vi "InitializePicomotor8742Controller.vi"(8 "error in (no error)":errorcluster, 11 "Picomotor8742 in":refnum<class "Picomotor8742.lvclass">) -> (0 "error out":errorcluster, 3 "Picomotor8742 out":refnum<class "Picomotor8742.lvclass">)   [LabVIEW 2020, in "Picomotor8742.lvclass"]
doc: "Initialize the class \"Picomotor8742ControllerClass\" that handles the communication with the physical device , and open the communication with the device"
uses:
  Picomotor8742.lvclass
  SupportLibs/TCPCommClass/TCPCommClass.lvclass
  C:/GEECS/Developers Version/source/Device Drivers/Picomotor8742/SupportLibs/ASCIICommClass/ASCIICommClass.lvclass
  SupportLibs/PicoMotorController/Picomoto8742ControllerClass.lvclass
  SupportLibs/PicoMotor8472Comm/PicoMotor8742Comm.lvclass
  Picomotor8742.lvclass/Picomotor8742.ctl
  SupportLibs/PicoMotor8742Axis/Picomotor8742Axis.lvclass
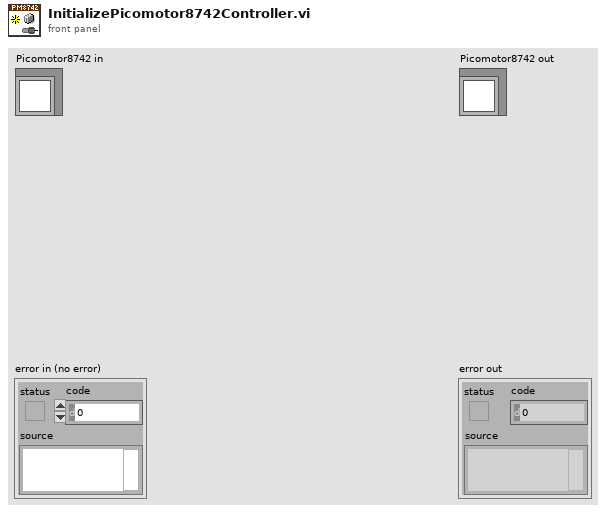
[diagram p1: front panel]
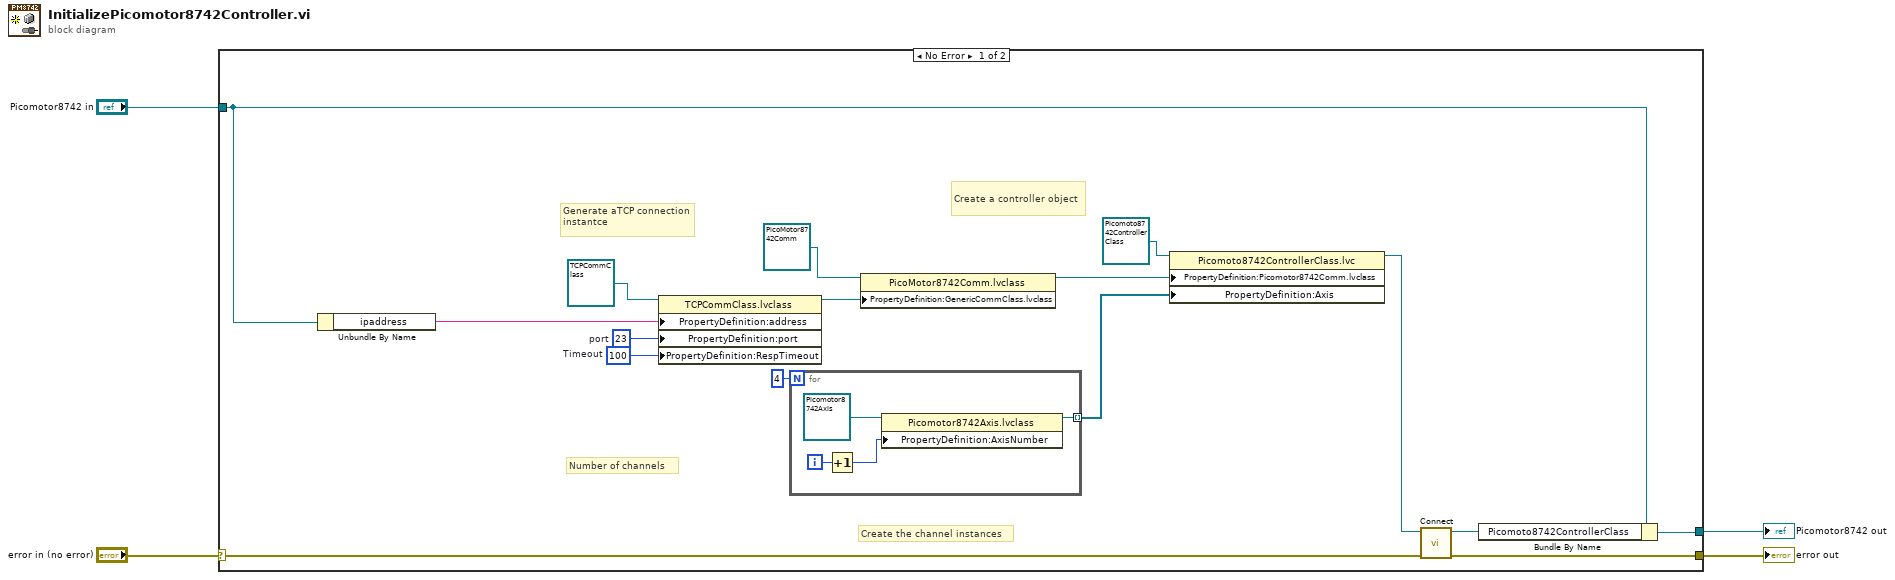
[diagram p0: block diagram]
diagram:
  n1 = case shown="No Error" "error in (no error)" {
    selector: "error in (no error)" -> [w9 w26]
    tunnel: [w8 w26] -> w3
    tunnel: [w5 w25] -> w1
    tunnel: "Picomotor8742 in" -> [w6 w25]
    frame No Error {
      w18 = u16 100  # Timeout
      w19 = u16 23  # port
      # "Create a controller object"
      # "Number of channels"
      # "Generate aTCP connection instantce"
      # "Create the channel instances"
      n2 = Unbundle By Name(w6) -> ("ipaddress"=w13:string)
      n3 = property class="TCPCommClass.lvclass"(reference=refnum<class "TCPCommClass.lvclass"> refnum ("Picomotor8742Comm in"), "PropertyDefinition:address"=w13, "PropertyDefinition:port"=w19, "PropertyDefinition:RespTimeout"=w18) -> (reference out=w16:refnum<class "TCPCommClass.lvclass">)  [unwired: 1 in, 1 out]
      n4 = for {
        N: 4 -> [_]
        tunnel: [w21] -> w11 mode=indexing
        i -> [w22]
        n5 = Increment(x=w22) -> (x+1=w23:i32)
        n6 = property class="Picomotor8742Axis.lvclass"(reference=refnum<class "Picomotor8742Axis.lvclass"> refnum ("Picomotor8742Axis.lvclass"), "PropertyDefinition:AxisNumber"=w23) -> (reference out=w21:refnum<class "Picomotor8742Axis.lvclass">)  [unwired: 1 in, 1 out]
      }
      n7 = property class="PicoMotor8742Comm.lvclass"(reference=refnum<class "PicoMotor8742Comm.lvclass"> refnum ("PicoMotor8742Comm.lvclass"), "PropertyDefinition:GenericCommClass.lvclass"=w16) -> (reference out=w15:refnum<class "PicoMotor8742Comm.lvclass">)  [unwired: 1 in, 1 out]
      n8 = property class="Picomoto8742ControllerClass.lvc"(reference=refnum<class "Picomoto8742ControllerClass.lvclass"> refnum ("Picomoto8742ControllerClass.lvclass"), "PropertyDefinition:Picomotor8742Comm.lvclass"=w15, "PropertyDefinition:Axis"=w11) -> (reference out=w14:refnum<class "Picomoto8742ControllerClass.lvclass">)  [unwired: 1 in, 1 out]
      n9 = call-dynamic "Connect.vi"("error in (no error)"=w9, "Picomoto8742ControllerClass in"=w14) -> ("error out"=w8:errorcluster, "Picomoto8742ControllerClass out"=w7:refnum<class "Picomoto8742ControllerClass.lvclass">)  [unwired: 8 in]
      n10 = Bundle By Name(cluster=w6, "Picomoto8742ControllerClass"=w7) -> (w5:refnum<class "Picomotor8742.lvclass">)
    }
    frame Error {
    }
  }
  "error out" <- w3
  "Picomotor8742 out" <- w1
